vi "BAOCAOTDO.vi"() -> ()   [LabVIEW 2024]
panel:
  in  "motor 3":bool
  in  "motor 2":bool
  in  "motor 1":bool
  out "sensor3":string
  out "sensor2":string
  out "sensor1":string
  out "sensor 1":dbl(slide) scale=0.0..100.0
  out "sensor 2":dbl(slide) scale=0.0..100.0
  out "sensor 3":dbl(slide) scale=0.0..100.0
  out "HIGH":bool
  out "MEDIUM":bool
  out "LOW":bool
  # "GIAM SAT MUC NUOC"
  # "ALARM:"
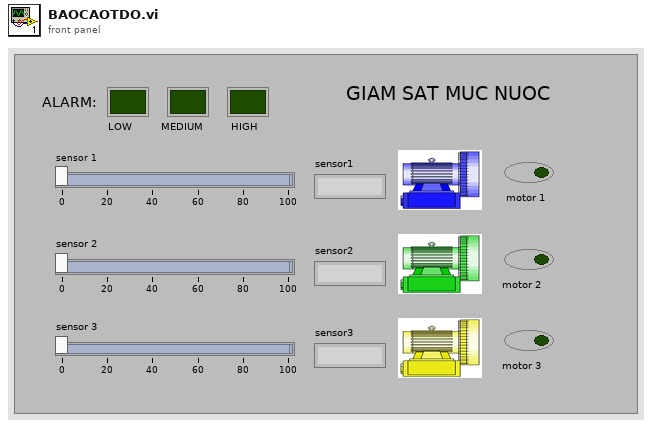
[diagram p1: front panel]
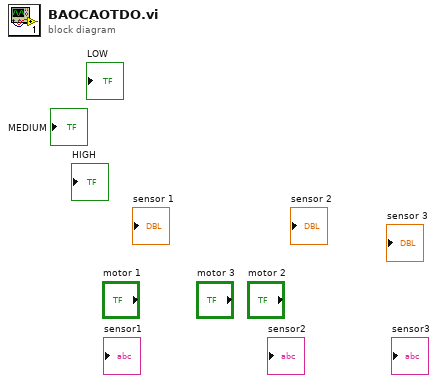
[diagram p0: block diagram]
diagram:
